vi "LC ControlPath.vi"(6 "Parent Tag":string, 8 "error in (no error)":errorcluster caption="Error In", 9 "Treeref":refnum<vi>, 10 "Control Path In":string, 11 "Ctl Ref In":refnum<vi>) -> (0 "error out":errorcluster caption="Error Out", 2 "Control Path Out":string[](array[string]), 3 "Ctl Ref Out":refnum<vi>[](array[refnum]))   [LabVIEW 2020]
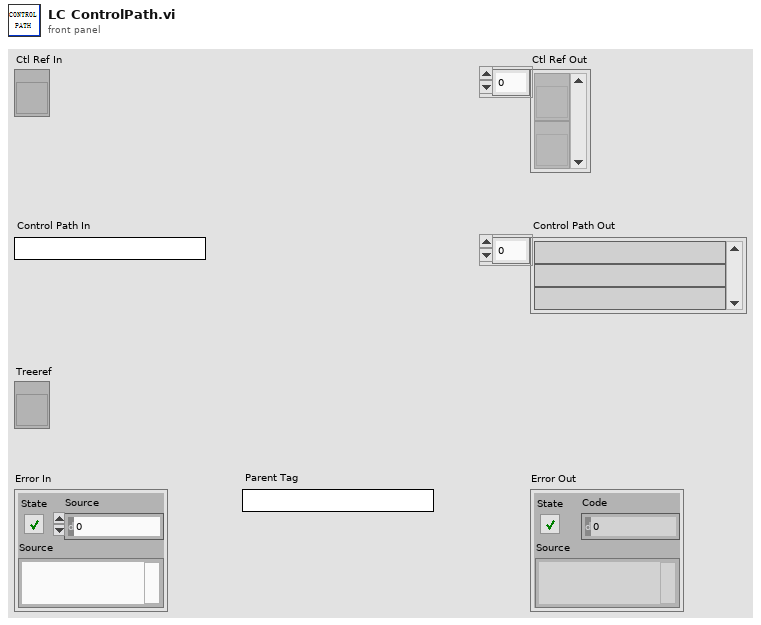
[diagram p1: front panel]
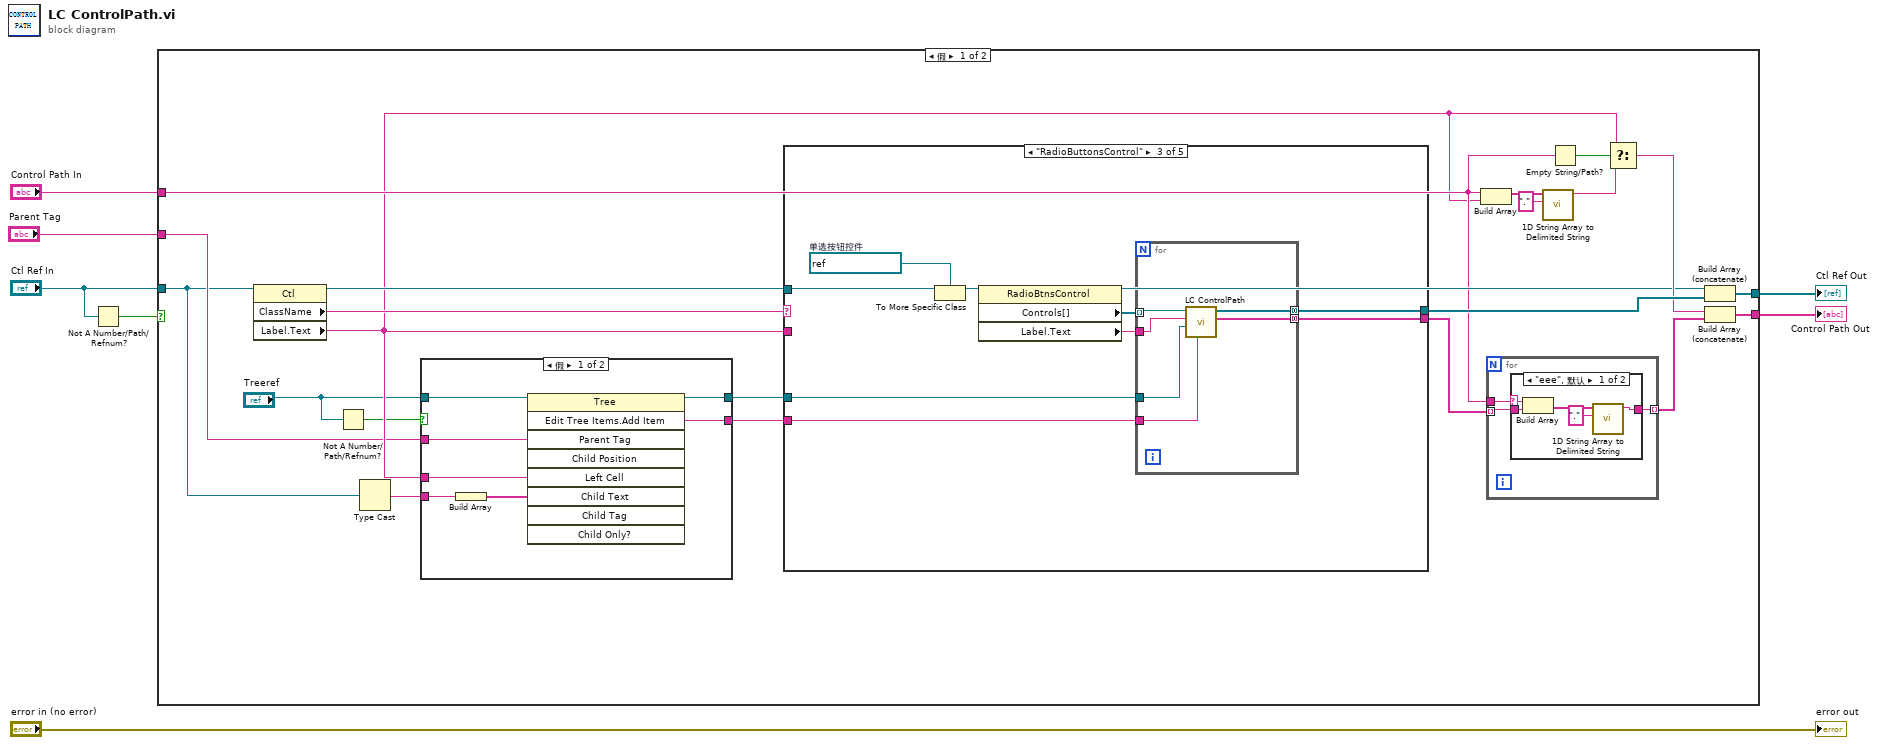
[diagram p0: block diagram]
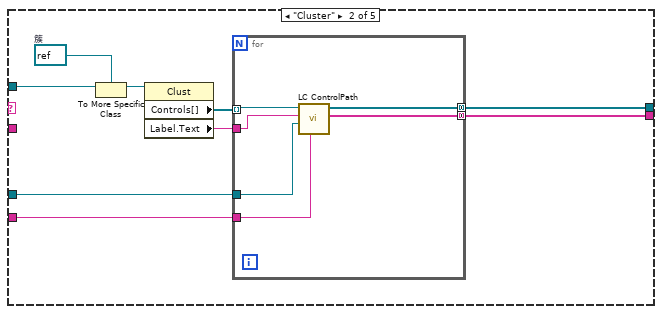
[diagram p5: hidden frame]
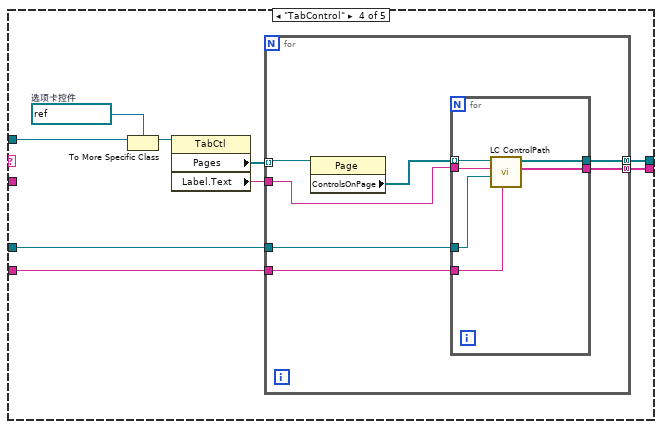
[diagram p6: hidden frame]
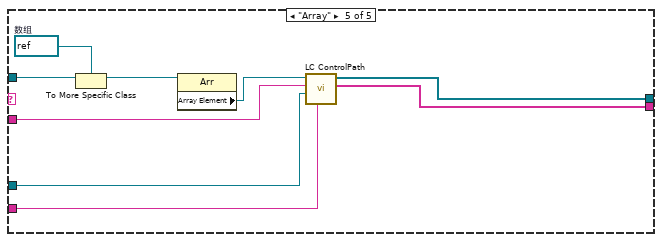
[diagram p7: hidden frame]
diagram:
  n1 = Not A Number/Path/Refnum?(number/path/refnum="Ctl Ref In") -> (NaN/Path/Refnum?=w5:bool)
  n2 = case shown="假" w5 {
    tunnel: "Ctl Ref In" -> [w8 _]
    tunnel: "Control Path In" -> [w16 _]
    tunnel: [w25 _] -> w3
    tunnel: [w23 _] -> w2
    tunnel: "Parent Tag" -> [w10 _]
    frame False {
      n3 = property class="Ctl"(reference=w8) -> (reference out=w19:refnum<vi>, "ClassName"=w28:string, "Label.Text"=w15:string)  [unwired: 1 in, 1 out]
      n4 = Not A Number/Path/Refnum?(number/path/refnum="Treeref") -> (NaN/Path/Refnum?=w12:bool)
      n5 = Type Cast(x=w8) -> (*(type *) &x=w9:string)  [unwired: 1 in]
      n6 = case shown="假" w12 {
        tunnel: w10 -> [w35 w36]
        tunnel: w15 -> [w34 _]
        tunnel: [w33 w36] -> w14
        tunnel: [w32 w37] -> w13
        tunnel: "Treeref" -> [w31 w37]
        tunnel: w9 -> [w30 _]
        frame False {
          n7 = Build Array(w30) -> (w29:string[])
          n8 = invoke class="Tree" method="Edit Tree Items.Add Item"(reference=w31, "Parent Tag"=w35, "Left Cell"=w34, "Child Text"=w29) -> (reference out=w32:refnum<vi>, "Edit Tree Items:Add Item"=w33:string)  [unwired: 5 in, 7 out]
        }
        frame True {
        }
      }
      n9 = case shown="\"RadioButtonsControl\"" w28 {
        tunnel: [_ w50 w66 w80 w105] -> w18
        tunnel: w19 -> [_ w55 w70 w85 w104]
        tunnel: [_ w49 w65 w79 w106] -> w24
        tunnel: w15 -> [_ _ _ _ w107]
        tunnel: w14 -> [_ w48 w63 w78 w100]
        tunnel: w13 -> [_ w47 w62 w77 w99]
        frame "eee", Default {
        }
        frame "Cluster" {
          w54 = refnum<vi> refnum  # 簇
          n10 = To More Specific Class(target class=w54, reference=w55) -> (specific class reference=w53:refnum<vi>)  [unwired: 1 in, 1 out]
          n11 = property class="Clust"(reference=w53) -> ("Controls[]"=w52:refnum<vi>[], "Label.Text"=w51:string)  [unwired: 1 in, 2 out]
          n12 = for {
            tunnel: w52 -> [w61] mode=indexing
            tunnel: w51 -> [w58]
            tunnel: [w60] -> w50 mode=concatenating
            tunnel: [w59] -> w49 mode=concatenating
            tunnel: w48 -> [w57]
            tunnel: w47 -> [w56]
            n13 = call "LC ControlPath.vi"("Parent Tag"=w57, "Treeref"=w56, "Control Path In"=w58, "Ctl Ref In"=w61) -> ("Control Path Out"=w60:string[], "Ctl Ref Out"=w59:refnum<vi>[])  [unwired: 5 in, 1 out]
          }
        }
        frame "RadioButtonsControl" {
          w64 = refnum<vi> refnum  # 单选按钮控件
          n14 = To More Specific Class(target class=w64, reference=w70) -> (specific class reference=w69:refnum<vi>)  [unwired: 1 in, 1 out]
          n15 = property class="RadioBtnsControl"(reference=w69) -> ("Controls[]"=w68:refnum<vi>[], "Label.Text"=w67:string)  [unwired: 1 in, 2 out]
          n16 = for {
            tunnel: w68 -> [w76] mode=indexing
            tunnel: w67 -> [w73]
            tunnel: [w75] -> w66 mode=concatenating
            tunnel: [w74] -> w65 mode=concatenating
            tunnel: w63 -> [w72]
            tunnel: w62 -> [w71]
            n17 = call "LC ControlPath.vi"("Parent Tag"=w72, "Treeref"=w71, "Control Path In"=w73, "Ctl Ref In"=w76) -> ("Control Path Out"=w75:string[], "Ctl Ref Out"=w74:refnum<vi>[])  [unwired: 5 in, 1 out]
          }
        }
        frame "TabControl" {
          w84 = refnum<vi> refnum  # 选项卡控件
          n18 = To More Specific Class(target class=w84, reference=w85) -> (specific class reference=w83:refnum<vi>)  [unwired: 1 in, 1 out]
          n19 = property class="TabCtl"(reference=w83) -> ("Pages"=w82:refnum<vi>[], "Label.Text"=w81:string)  [unwired: 1 in, 2 out]
          n20 = for {
            tunnel: w82 -> [w92] mode=indexing
            tunnel: w81 -> [w88]
            tunnel: [w91] -> w80 mode=concatenating
            tunnel: [w90] -> w79 mode=concatenating
            tunnel: w78 -> [w87]
            tunnel: w77 -> [w86]
            n21 = property class="Page"(reference=w92) -> ("ControlsOnPage"=w89:refnum<vi>[])  [unwired: 1 in, 2 out]
            n22 = for {
              tunnel: w89 -> [w98] mode=indexing
              tunnel: [w97] -> w91
              tunnel: [w96] -> w90
              tunnel: w88 -> [w95]
              tunnel: w87 -> [w94]
              tunnel: w86 -> [w93]
              n23 = call "LC ControlPath.vi"("Parent Tag"=w94, "Treeref"=w93, "Control Path In"=w95, "Ctl Ref In"=w98) -> ("Control Path Out"=w97:string[], "Ctl Ref Out"=w96:refnum<vi>[])  [unwired: 5 in, 1 out]
            }
          }
        }
        frame "Array" {
          w103 = refnum<vi> refnum  # 数组
          n24 = To More Specific Class(target class=w103, reference=w104) -> (specific class reference=w102:refnum<vi>)  [unwired: 1 in, 1 out]
          n25 = property class="Arr"(reference=w102) -> ("Array Element"=w101:refnum<vi>)  [unwired: 1 in, 2 out]
          n26 = call "LC ControlPath.vi"("Parent Tag"=w100, "Treeref"=w99, "Control Path In"=w107, "Ctl Ref In"=w101) -> ("Control Path Out"=w105:string[], "Ctl Ref Out"=w106:refnum<vi>[])  [unwired: 5 in, 1 out]
        }
      }
      n27 = Build Array(w16, w15) -> (w27:string[])
      n28 = for {
        tunnel: w18 -> [w39] mode=indexing
        tunnel: w16 -> [w40]
        tunnel: [w38] -> w17 mode=indexing
        n29 = case shown="\"eee\", 默认" w40 {
          selector: w40 -> [w44 _]
          tunnel: w39 -> [w43 w46]
          tunnel: [w41 w46] -> w38
          frame "eee", Default {
            n30 = Build Array(w44, w43) -> (w42:string[])
            n31 = call <vilib>:"1D String Array to Delimited String.vi"("delimiter"=".", "string array"=w42) -> ("delimited string"=w41:string)  [unwired: 9 in]
          }
          frame "" {
          }
        }
      }
      n32 = call <vilib>:"1D String Array to Delimited String.vi"("delimiter"=".", "string array"=w27) -> ("delimited string"=w21:string)  [unwired: 9 in]
      n33 = Empty String/Path?(string/path=w16) -> (empty?=w22:bool)
      n34 = Select(t=w15, s=w22, f=w21) -> (s? t:f=w20:string)
      n35 = Build Array (concatenate)(w19, w24) -> (w23:refnum<vi>[])
      n36 = Build Array (concatenate)(w20, w17) -> (w25:string[])
    }
    frame True {
    }
  }
  "Control Path Out" <- w3
  "Ctl Ref Out" <- w2
  "error out" <- "error in (no error)"
